vi "ER2007 Current Values Panel.vi"() -> ()   [LabVIEW 2013]
uses:
  Controls/Global ER2007.vi
panel:
  out "Pc5Xdcr":string="Pore Press (Hi)"
  out "Pc4Xdcr":string="Pore Press (Hi)"
  out "Pc3Xdcr":string="Pore Press (Hi)"
  out "Pc2Xdcr":string="Pore Press (Hi)"
  out "Pc1Xdcr":string="Pore Press (Hi)"
  out "Title 5":string="Cell 5"
  out "Title 4":string="Cell 4"
  out "Title 3":string="Cell 3"
  out "Title 2":string="Cell 2"
  out "Title 1":string="Cell 1"
  out "Pvol 5":dbl=3504.1 format="%.2f"
  out "Pdp 5":dbl=3504.1 format="%.2f"
  out "Pvol 4":dbl=3504.1 format="%.2f"
  out "Pdp 4":dbl=3504.1 format="%.2f"
  out "Pvol 3":dbl=3504.1 format="%.2f"
  out "Pdp 3":dbl=3504.1 format="%.2f"
  out "Pvol 2":dbl=3504.1 format="%.2f"
  out "Pdp 2":dbl=3504.1 format="%.2f"
  out "Pvol 1":dbl=3504.1 format="%.2f"
  out "Pdp 1":dbl=3504.1 format="%.2f"
  in  "Exit":bool
  out "Pc 5":dbl=2211.4
  out "NOP 5":dbl=2993.8
  out "TB 5":dbl=65.1 format="%.1f"
  out "TA 5":dbl=65.6 format="%.1f"
  out "Pc 4":dbl=0.9
  out "NOP 4":dbl
  out "TB 4":dbl=22.6 format="%.1f"
  out "TA 4":dbl=22.4 format="%.1f"
  out "Pc 3":dbl=3488.6
  out "NOP 3":dbl=5026.3
  out "TB 3":dbl=75.1 format="%.1f"
  out "TA 3":dbl=74.9 format="%.1f"
  out "Pc 2":dbl=-0.6
  out "NOP 2":dbl=0.3
  out "TB 2":dbl=22.5 format="%.1f"
  out "TA 2":dbl=22.8 format="%.1f"
  out "Pc 1":dbl=3504.1
  out "NOP 1":dbl=5013.7
  out "TB 1":dbl=75.0 format="%.1f"
  out "TA 1":dbl=75.3 format="%.1f"
  # "Cell Current Values"
  # "Temp A"
  # "Temp A"
  # "Temp A"
  # "Temp A"
  # "Temp A"
  # "(C)"
  # "(C)"
  # "(C)"
  # "(C)"
  # "(C)"
  # "Temp B"
  # "Temp B"
  # "Temp B"
  # "Temp B"
  # "Temp B"
  # "(C)"
  # "(C)"
  # "(C)"
  # "(C)"
  # "(C)"
  # "Conf Press"
  # "Conf Press"
  # "Conf Press"
  # "Conf Press"
  # "Conf Press"
  # "(psi)"
  # "(psi)"
  # "(psi)"
  # "(psi)"
  # "(psi)"
  # "(psi)"
  # "(psi)"
  # "(psi)"
  # "(psi)"
  # "(psi)"
  # "Delta-P"
  # "Delta-P"
  # "Delta-P"
  # "Delta-P"
  # "Delta-P"
  # "(psi)"
  # "(psi)"
  # "(psi)"
  # "(psi)"
  # "(psi)"
  # "Produced Vol"
  # "Produced Vol"
  # "Produced Vol"
  # "Produced Vol"
  # "Produced Vol"
  # "(ml)"
  # "(ml)"
  # "(ml)"
  # "(ml)"
  # "(ml)"
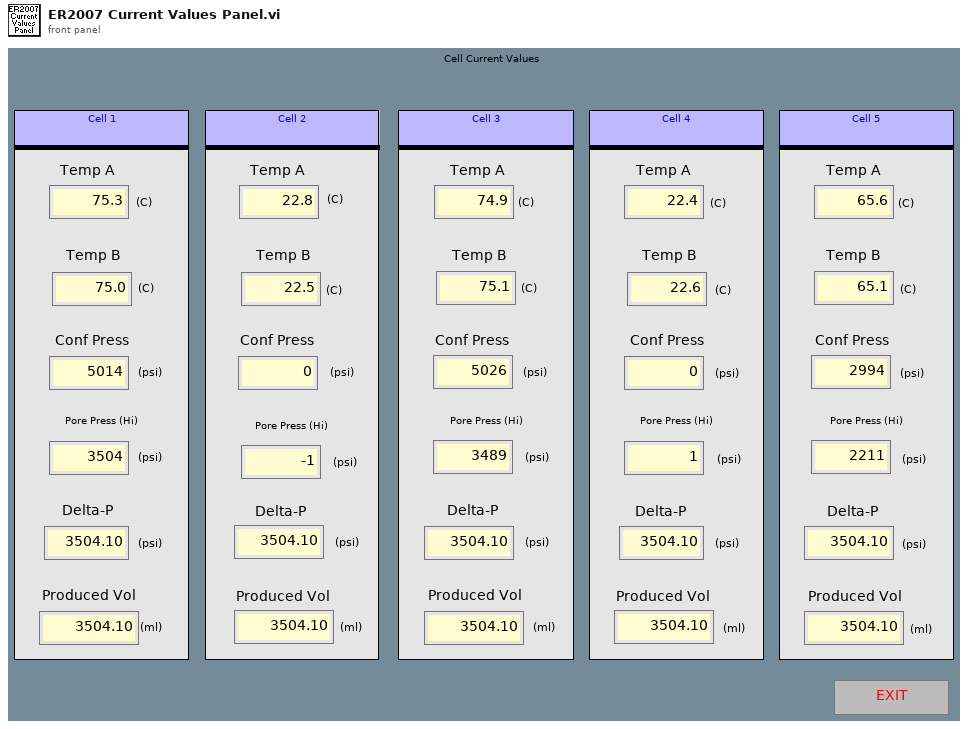
[diagram p1: front panel]
types:
  T1 = cluster{"CurCell":i32, "Cell Data":cluster{"Cell ID":i32, "Cell Status":enum16{"Inactive", "Setup", "Active", "Done"}, "Project":string, "Sample #":string, "Rock Type":string, "Fluid Pair":string, "Rw":dbl, "Rw Temp":dbl, "Length":dbl, "Diameter":dbl, "Porosity":dbl, "Permeability":dbl, "4P":bool, "ElectSpace":dbl, "Frequency":dbl, "Amplitude":dbl, "DAQ Period":u32, "DAQ Units":u16, "Start Time":dbl, "Next Time":dbl, "Datafile":path, "Last Pore Vol":dbl, "Last Pore Xdcr":enum16{"<none>", "Lo Range", "Hi Range"}, "Last Resistor":enum16{"<none>", "Resistor 1", "Resistor 2", "Resistor 3", "Resistor 4", "Resistor 5", "Resistor 6"}, "CurData":dbl[][], "Comment":string}[]}
  T2 = cluster{"Cell ID":i32, "Cell Status":enum16{"Inactive", "Setup", "Active", "Done"}, "Project":string, "Sample #":string, "Rock Type":string, "Fluid Pair":string, "Rw":dbl, "Rw Temp":dbl, "Length":dbl, "Diameter":dbl, "Porosity":dbl, "Permeability":dbl, "4P":bool, "ElectSpace":dbl, "Frequency":dbl, "Amplitude":dbl, "DAQ Period":u32, "DAQ Units":u16, "Start Time":dbl, "Next Time":dbl, "Datafile":path, "Last Pore Vol":dbl, "Last Pore Xdcr":enum16{"<none>", "Lo Range", "Hi Range"}, "Last Resistor":enum16{"<none>", "Resistor 1", "Resistor 2", "Resistor 3", "Resistor 4", "Resistor 5", "Resistor 6"}, "CurData":dbl[][], "Comment":string}[]
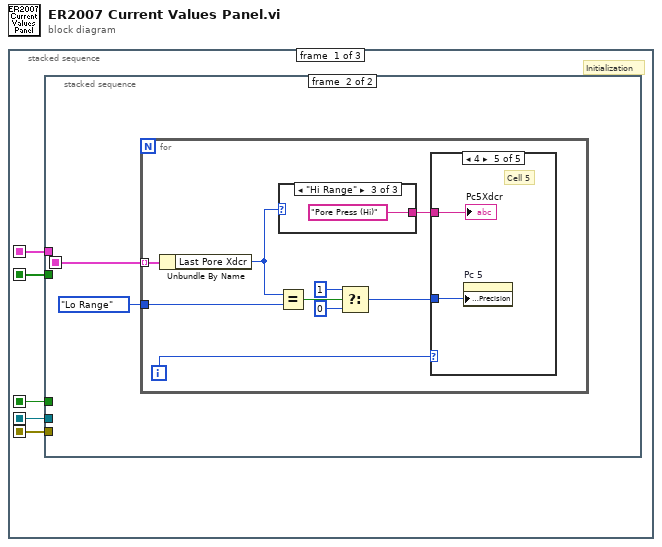
[diagram p0: block diagram]
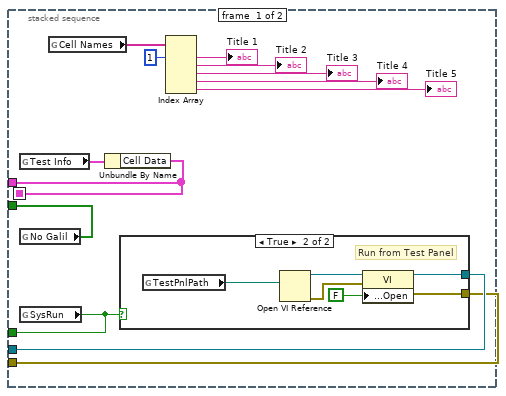
[diagram p2: hidden frame]
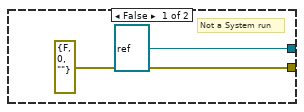
[diagram p3: hidden frame]
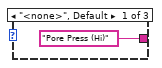
[diagram p4: hidden frame]
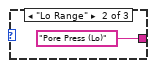
[diagram p5: hidden frame]
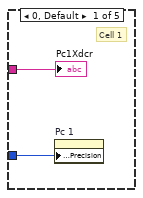
[diagram p6: hidden frame]
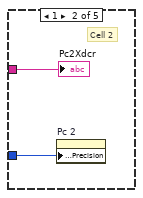
[diagram p7: hidden frame]
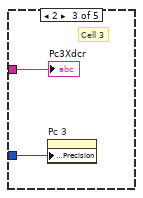
[diagram p8: hidden frame]
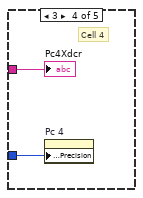
[diagram p9: hidden frame]
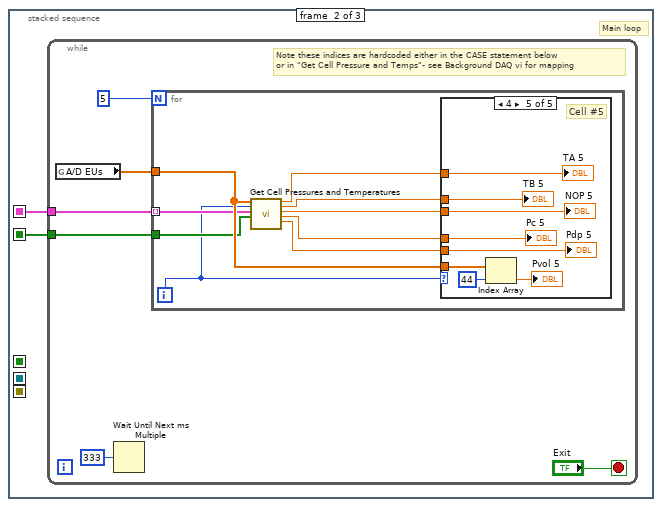
[diagram p10: hidden frame]
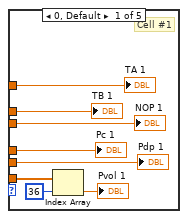
[diagram p11: hidden frame]
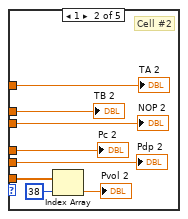
[diagram p12: hidden frame]
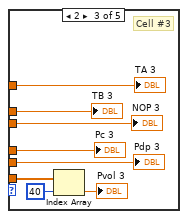
[diagram p13: hidden frame]
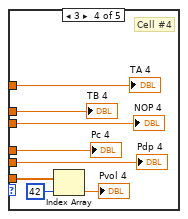
[diagram p14: hidden frame]
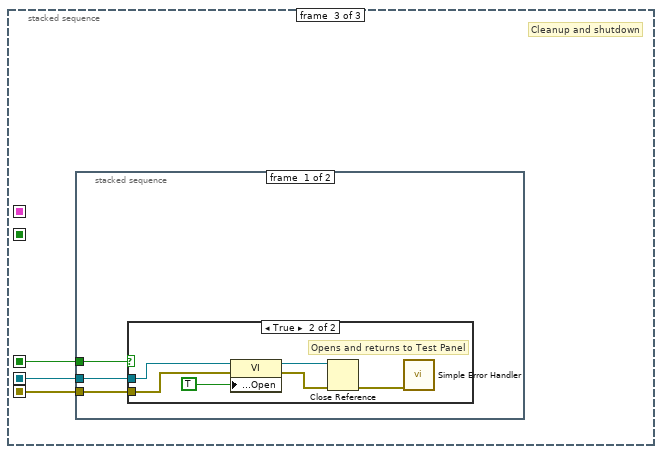
[diagram p15: hidden frame]
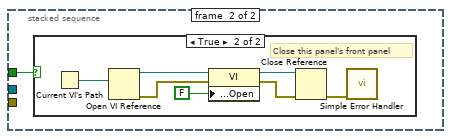
[diagram p17: hidden frame]
diagram:
  n1 = stacked-sequence {
    seq-local: [w5 _ _] -> [_ _ w110]
    seq-local: [w4 _ _] -> [_ _ w109]
    seq-local: [w3 _ _] -> [_ _ w108]
    seq-local: [w2 _ _] -> [_ w52 _]
    seq-local: [w1 _ _] -> [_ w51 _]
    frame #0 {
      # "Initialization"
      n2 = stacked-sequence {
        seq-local: [w6 _] -> [_ w28]
        tunnel: [w16 _] -> w5
        tunnel: [w18 _] -> w4
        tunnel: [w17 _] -> w3
        tunnel: [w8 _] -> w2
        tunnel: [w6 _] -> w1
        frame #0 {
          n3 = global read "Global ER2007.vi" "Test Info"() -> (w7:T1)
          n4 = global read "Global ER2007.vi" "No Galil"() -> (w8:bool[])
          n5 = global read "Global ER2007.vi" "SysRun"() -> (w16:bool)
          n6 = global read "Global ER2007.vi" "Cell Names"() -> (w15:string[])
          n7 = Unbundle By Name(w7) -> ("Cell Data"=w6:T2)
          n8 = case shown="True" w16 {
            tunnel: [refnum<vi> refnum w23] -> w18
            tunnel: [errorcluster {"status"=FALSE, "code"=0, "source"=""} ("error out") w22] -> w17
            frame False {
              # "Not a System run"
            }
            frame True {
              # "Run from Test Panel"
              n9 = global read "Global ER2007.vi" "TestPnlPath"() -> (w21:path)
              n10 = Open VI Reference(vi path=w21) -> (vi reference=w26:refnum<vi>, error out=w25:errorcluster)  [unwired: 5 in]
              n11 = property class="VI"(reference=w26, error in=w25, "Front Panel Window:Open"=FALSE) -> (reference out=w23:refnum<vi>, error out=w22:errorcluster)
            }
          }
          n12 = Index Array(array=w15, index #1=1 ("index")) -> (element #1=→"Title 1":string, element #2=→"Title 2":string, element #3=→"Title 3":string, element #4=→"Title 4":string, element #5=→"Title 5":string)  [unwired: 4 in]
        }
        frame #1 {
          n13 = for {
            tunnel: w28 -> [w37] mode=indexing
            tunnel: enum16{"<none>", "Lo Range", "Hi Range"}."Lo Range" ("Last Pore Xdcr") -> [w32]
            i -> [w36]
            n14 = Unbundle By Name(w37) -> ("Last Pore Xdcr"=w31:enum16{"<none>", "Lo Range", "Hi Range"})
            n15 = Equal?(x=w31, y=w32) -> (x = y?=w35:bool)
            n16 = case shown="\"Hi Range\"" w31 {
              tunnel: ["Pore Press (Hi)" "Pore Press (Lo)" "Pore Press (Hi)"] -> w30
              frame "<none>", Default {
              }
              frame "Lo Range" {
              }
              frame "Hi Range" {
              }
            }
            n17 = Select(t=u8 1 ("Format & Precision:Precision"), s=w35, f=u8 0 ("Format & Precision:Precision")) -> (s? t:f=w29:u8)
            n18 = case shown="4" w36 {
              tunnel: w30 -> [w42 w43 w46 w48 w50]
              tunnel: w29 -> [w41 w44 w45 w47 w49]
              frame 0, Default {
                # "Cell 1"
                n19 = property on="Pc 1" class="DigNum (strict)"("Display Format:Precision"=w41) -> ()  [unwired: 2 in, 2 out]
                "Pc1Xdcr" <- w42
              }
              frame 1 {
                # "Cell 2"
                n20 = property on="Pc 2" class="DigNum (strict)"("Display Format:Precision"=w44) -> ()  [unwired: 2 in, 2 out]
                "Pc2Xdcr" <- w43
              }
              frame 2 {
                # "Cell 3"
                n21 = property on="Pc 3" class="DigNum (strict)"("Display Format:Precision"=w45) -> ()  [unwired: 2 in, 2 out]
                "Pc3Xdcr" <- w46
              }
              frame 3 {
                # "Cell 4"
                n22 = property on="Pc 4" class="DigNum (strict)"("Display Format:Precision"=w47) -> ()  [unwired: 2 in, 2 out]
                "Pc4Xdcr" <- w48
              }
              frame 4 {
                # "Cell 5"
                n23 = property on="Pc 5" class="DigNum (strict)"("Display Format:Precision"=w49) -> ()  [unwired: 2 in, 2 out]
                "Pc5Xdcr" <- w50
              }
            }
          }
        }
      }
    }
    frame #1 {
      # "Main loop"
      n24 = while {
        tunnel: w52 -> [w54]
        tunnel: w51 -> [w53]
        stop <- "Exit" stop-if-true
        # "Note these indices are hardcoded either in the CASE statement below\nor in \"Get Cell Pressure and Temps\"- see Background DAQ vi for mapping"
        n25 = global read "Global ER2007.vi" "A/D EUs"() -> (w56:dbl[])
        n26 = Wait Until Next ms Multiple(millisecond multiple=u32 333) -> ()  [unwired: 1 out]
        n27 = for {
          N: 5 -> [_]
          tunnel: w56 -> [w67]
          tunnel: w54 -> [w61]
          tunnel: w53 -> [w60] mode=indexing
          i -> [w59]
          n28 = call "Get Cell Pressures and Temperatures.vi"("EUs"=w67, "Cell #"=w59, "Cell x Data"=w60, "No Galil"=w61) -> ("T-A"=w66:dbl, "T-B"=w65:dbl, "NOP"=w64:dbl, "Pc"=w63:dbl, "Delta-P"=w62:dbl)  [unwired: 10 in, 1 out]
          n29 = case shown="4" w59 {
            tunnel: w67 -> [w74 w77 w85 w93 w101]
            tunnel: w62 -> [w73 w79 w87 w95 w103]
            tunnel: w63 -> [w72 w80 w88 w96 w104]
            tunnel: w64 -> [w71 w81 w89 w97 w105]
            tunnel: w65 -> [w70 w82 w90 w98 w106]
            tunnel: w66 -> [w69 w83 w91 w99 w107]
            frame 0, Default {
              # "Cell #1"
              n30 = Index Array(array=w74, index=36) -> (element=→"Pvol 1":dbl)
              "TA 1" <- w69
              "TB 1" <- w70
              "NOP 1" <- w71
              "Pc 1" <- w72
              "Pdp 1" <- w73
            }
            frame 1 {
              # "Cell #2"
              n31 = Index Array(array=w77, index=38) -> (element=→"Pvol 2":dbl)
              "TA 2" <- w83
              "TB 2" <- w82
              "NOP 2" <- w81
              "Pc 2" <- w80
              "Pdp 2" <- w79
            }
            frame 2 {
              # "Cell #3"
              n32 = Index Array(array=w85, index=40) -> (element=→"Pvol 3":dbl)
              "TA 3" <- w91
              "TB 3" <- w90
              "NOP 3" <- w89
              "Pc 3" <- w88
              "Pdp 3" <- w87
            }
            frame 3 {
              # "Cell #4"
              n33 = Index Array(array=w93, index=42) -> (element=→"Pvol 4":dbl)
              "TA 4" <- w99
              "TB 4" <- w98
              "NOP 4" <- w97
              "Pc 4" <- w96
              "Pdp 4" <- w95
            }
            frame 4 {
              # "Cell #5"
              n34 = Index Array(array=w101, index=44) -> (element=→"Pvol 5":dbl)
              "TA 5" <- w107
              "TB 5" <- w106
              "NOP 5" <- w105
              "Pc 5" <- w104
              "Pdp 5" <- w103
            }
          }
        }
      }
    }
    frame #2 {
      # "Cleanup and shutdown"
      n35 = stacked-sequence {
        tunnel: w110 -> [w111 w120]
        tunnel: w109 -> [w113 _]
        tunnel: w108 -> [w112 _]
        frame #0 {
          n36 = case shown="True" w111 {
            tunnel: w113 -> [_ w114]
            tunnel: w112 -> [_ w115]
            frame False {
            }
            frame True {
              # "Opens and returns to Test Panel"
              n37 = property class="VI"(reference=w114, error in=w115, "Front Panel Window:Open"=TRUE) -> (reference out=w118:refnum<vi>, error out=w117:errorcluster)
              n38 = Close Reference(reference=w118, error in (no error)=w117) -> (error out=w116:errorcluster)
              n39 = call <vilib>:"Simple Error Handler.vi"("error in (no error)"=w116) -> ()  [unwired: 4 in, 5 out]
            }
          }
        }
        frame #1 {
          n40 = case shown="True" w120 {
            frame False {
            }
            frame True {
              # "Close this panel's front panel"
              n41 = Current VI's Path() -> (path=w127:path)
              n42 = Open VI Reference(vi path=w127) -> (vi reference=w126:refnum<vi>, error out=w125:errorcluster)  [unwired: 5 in]
              n43 = property class="VI"(reference=w126, error in=w125, "Front Panel Window:Open"=FALSE) -> (reference out=w123:refnum<vi>, error out=w122:errorcluster)
              n44 = Close Reference(reference=w123, error in (no error)=w122) -> (error out=w121:errorcluster)
              n45 = call <vilib>:"Simple Error Handler.vi"("error in (no error)"=w121) -> ()  [unwired: 4 in, 5 out]
            }
          }
        }
      }
    }
  }
